vi "_Pull Controls Value to DPs(Refmgr).vi"(6 "sync DPs?(T)":bool=TRUE, 7 "VIRef(Caller VI)":refnum<k1>, 8 "error in (no error)":errorcluster, 9 "force update(F)":bool, 11 "SILAPI In":refnum<k1>) -> (0 "error out":errorcluster, 1 "Binded DPs":string[](array[string]), 3 "SILAPI Out":refnum<k1>)   [LabVIEW 2017, in "TagDB RefManager.lvlib"]
uses:
  TagDB RefManager.lvlib
  230c0da9-b6e4-44e0-8cb2-fe6bdec026ba.vi
  a90990ad-2366-4051-9646-140e847e3682.vi
  be640558-f0fc-44bb-96cd-108508b5fbdb.vi
  17cf8676-e257-4f33-957d-6af3ca117314.vi
  6c796322-1d76-4bdd-9aa2-7f47adde5471.vi
  024ec822-42c1-4cee-abf5-dbe2fbe4f70a.vi
  <userlib>/_NEVSTOP/TagDB/_Support/DataAccess/_NameCacher.vi
  <userlib>/_NEVSTOP/TagDB/_Support/Error/_[error50002]Invalid DataType.vi
  <userlib>/_NEVSTOP/TagDB/_Support/Error/_[error50000]Invalid DB REF.vi
  <userlib>/_NEVSTOP/TagDB/_Support/DataAccess/TagDB Ref to DVR.vi
  <userlib>/_NEVSTOP/TagDB/_Support/URL/TRIM-BOTH-SPACE.vi
  17cf8676-e257-4f33-957d-6af3ca117314.vi/1b47866c-8e2d-43a7-815f-8cf18635e5a1.vi
  6c796322-1d76-4bdd-9aa2-7f47adde5471.vi/1b47866c-8e2d-43a7-815f-8cf18635e5a1.vi
  <userlib>/_NEVSTOP/TagDB/_Support/DataAccess/data-Write.vi
  <userlib>/_NEVSTOP/TagDB/_Support/Change Detector/TagDB dbChanged.vi
  <userlib>/_NEVSTOP/TagDB/_Support/Error/_Clear Errors.vi
  17cf8676-e257-4f33-957d-6af3ca117314.vi/1b47866c-8e2d-43a7-815f-8cf18635e5a1.vi/29b2ea6d-6d7f-4e4a-ad31-a5cb760462c7.vi
  <userlib>/_NEVSTOP/TagDB/API/TagDB-Status.vi
  6c796322-1d76-4bdd-9aa2-7f47adde5471.vi/1b47866c-8e2d-43a7-815f-8cf18635e5a1.vi/29b2ea6d-6d7f-4e4a-ad31-a5cb760462c7.vi
  <userlib>/_NEVSTOP/TagDB/_Support/DataAccess/_datatypeChecker.vi
  <userlib>/_NEVSTOP/TagDB/_Support/Change Detector/TagDB ChangeFlag.vi
  <userlib>/_NEVSTOP/TagDB/_Support/Error/_Build Error Cluster.vi
  <vilib>/Utility/Data Type/Get Type Information.vi
  <userlib>/_NEVSTOP/TagDB/TagDB.lvlib
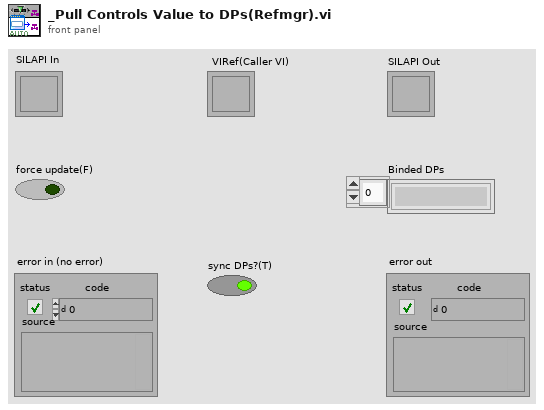
[diagram p1: front panel]
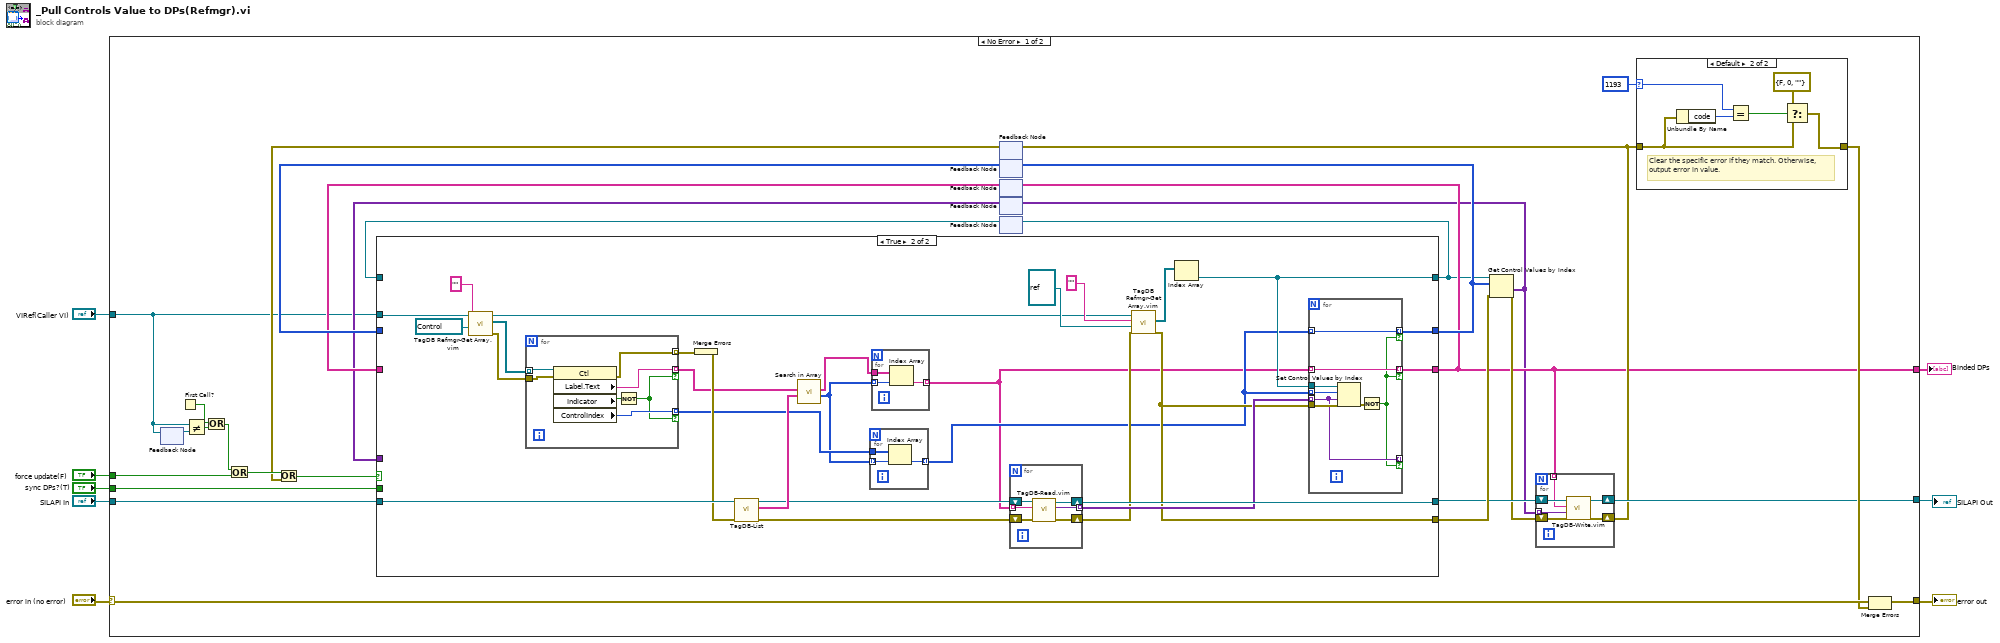
[diagram p0: block diagram]
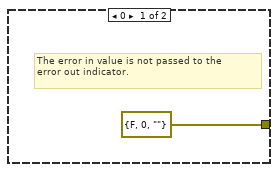
[diagram p2: hidden frame]
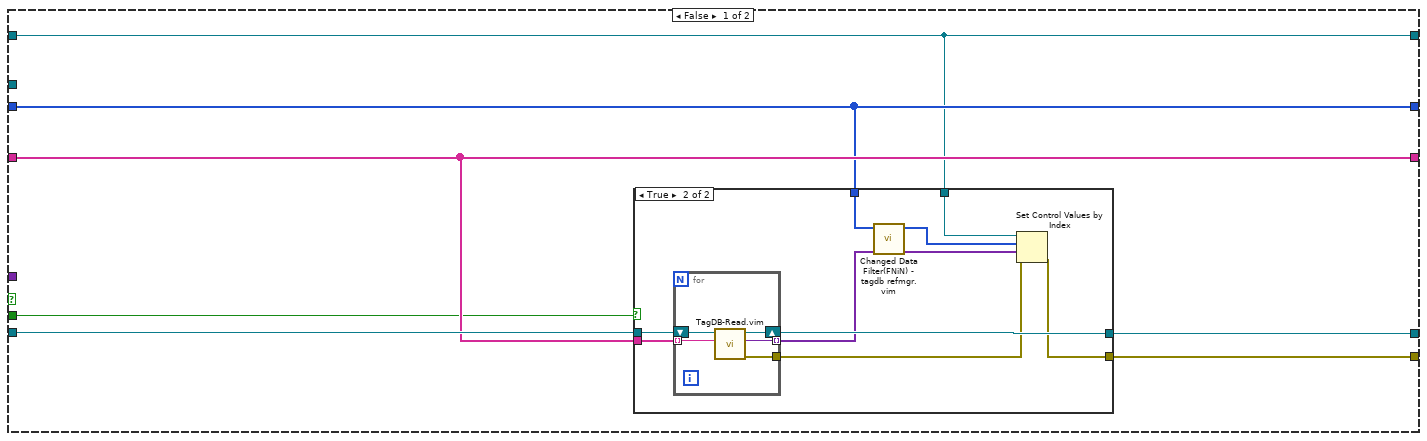
[diagram p3: hidden frame]
diagram:
  n1 = case shown="No Error" "error in (no error)" {
    selector: "error in (no error)" -> [w31 w129]
    tunnel: "force update(F)" -> [w36 _]
    tunnel: [w32 w129] -> w7
    tunnel: "SILAPI In" -> [w29 w128]
    tunnel: "VIRef(Caller VI)" -> [w9 _]
    tunnel: [w21 w128] -> w3
    tunnel: [w18 _] -> w2
    tunnel: "sync DPs?(T)" -> [w16 _]
    frame No Error {
      n2 = feedback #1() -> (w13:refnum<k1>)  [unwired: 1 in]
      n3 = feedback-in #1(w9) -> ()
      n4 = First Call?() -> (First Call?: T/F=w11:bool)
      n5 = Not Equal?(x=w9, y=w13) -> (x != y?=w12:bool)
      n6 = Or(x=w11, y=w12) -> (x .or. y?=w10:bool)
      n7 = Or(x=w10, y=w36) -> (x .or. y?=w33:bool)
      n8 = feedback #2() -> (w25:errorcluster)  [unwired: 1 in]
      n9 = Or(x=w33, y=w25) -> (x .or. y?=w26:bool)
      n10 = feedback #3() -> (w34:i32[])  [unwired: 1 in]
      n11 = feedback #4() -> (w30:string[])  [unwired: 1 in]
      n12 = feedback #5() -> (w28:variant[])  [unwired: 1 in]
      n13 = feedback #6() -> (w14:refnum<vi>)  [unwired: 1 in]
      n14 = case shown="True" w26 {
        tunnel: [w50 w80] -> w15
        tunnel: w9 -> [_ w88]
        tunnel: [w52 w95] -> w35
        tunnel: w34 -> [w52 _]
        tunnel: [w55 w96] -> w18
        tunnel: w30 -> [w55 _]
        tunnel: w29 -> [w56 w100]
        tunnel: [w53 w81] -> w23
        tunnel: w28 -> [_ _]
        tunnel: [w54 w98] -> w22
        tunnel: w16 -> [w51 _]
        tunnel: w14 -> [w50 _]
        frame False {
          n15 = case shown="True" w51 {
            tunnel: w56 -> [w57 w67]
            tunnel: w55 -> [_ w66]
            tunnel: [w57 w65] -> w54
            tunnel: w50 -> [_ w64]
            tunnel: [_ w62] -> w53
            tunnel: w52 -> [_ w59]
            frame False {
            }
            frame True {
              n16 = for {
                tunnel: w66 -> [w71] mode=indexing
                tunnel: [w69] -> w63
                tunnel: [w68] -> w61 mode=indexing
                shift-right: [w70] -> w65
                shift-left: w67 -> [w72]
                n17 = call "TagDB-Read.vim"("name"=w71, "TagDB"=w72) -> ("error out"=w69:errorcluster, "Value"=w68:variant, "TagDB(dup)"=w70:refnum<k1>)  [unwired: 4 in, 3 out]
              }
              n18 = call "Changed Data Filter(FNiN) - tagdb refmgr.vim"("checked data"=w61, "1"=w59) -> ("data"=w60:variant[], "1 out"=w58:i32[])  [unwired: 6 in, 2 out]
              n19 = Set Control Values by Index(0:w64, 1:w58, 2:w60, 3:w63) -> (11:w62:errorcluster)
            }
          }
        }
        frame True {
          n20 = call "TagDB Refmgr-Get Array.vim"("Type"=refnum<vi> refnum, "RegExp"="", "DB Ref"=w88) -> ("error out"=w87:errorcluster, "References"=w86:refnum<vi>[], "DB Ref(dup)"=w79:refnum<k1>)  [unwired: 5 in, 1 out]
          n21 = for {
            tunnel: w86 -> [w119] mode=indexing
            tunnel: [w118] -> w75 mode=indexing if=w113
            tunnel: [w117] -> w78 mode=indexing if=w113
            tunnel: [w115] -> w94 mode=indexing
            tunnel: w87 -> [w114]
            n22 = property class="Ctl"(reference=w119, error in=w114) -> (error out=w115:errorcluster, "Label.Text"=w118:string, "Indicator"=w116:bool, "ControlIndex"=w117:i32)  [unwired: 1 out]
            n23 = Not(x=w116) -> (.not. x?=w113:bool)
          }
          n24 = Merge Errors(w94) -> (w93:errorcluster)
          n25 = call <userlib>:"TagDB-List.vi"("error in (no error)"=w93, "TagDB"=w100) -> ("error out"=w99:errorcluster, "names"=w92:string[], "TagDB(dup)"=w91:refnum<k1>)  [unwired: 6 in, 1 out]
          n26 = call "Search in Array.vi"("items to filter"=w92, "array"=w75) -> ("item Indexs"=w76:i32[], "array(dup)"=w73:string[])  [unwired: 4 in]
          n27 = for {
            tunnel: w76 -> [w106] mode=indexing
            tunnel: w78 -> [w105]
            tunnel: [w104] -> w77 mode=indexing
            n28 = Index Array(array=w105, index=w106) -> (element=w104:i32)
          }
          n29 = for {
            tunnel: w76 -> [w103] mode=indexing
            tunnel: w73 -> [w102]
            tunnel: [w101] -> w74 mode=indexing
            n30 = Index Array(array=w102, index=w103) -> (element=w101:string)
          }
          n31 = for {
            tunnel: [w110] -> w97 mode=indexing
            tunnel: w74 -> [w108] mode=indexing
            shift-right: [w109] -> w82
            shift-left: w99 -> [w112]
            shift-right: [w111] -> w98
            shift-left: w91 -> [w107]
            n32 = call "TagDB-Read.vim"("error in (no error)"=w112, "name"=w108, "TagDB"=w107) -> ("error out"=w109:errorcluster, "Value"=w110:variant, "TagDB(dup)"=w111:refnum<k1>)  [unwired: 3 in, 3 out]
          }
          n33 = call "TagDB Refmgr-Get Array.vim"("error in (no error)"=w82, "Type"=refnum<vi> refnum ("Current VI Reference"), "RegExp"="", "DB Ref"=w79) -> ("error out"=w81:errorcluster, "References"=w83:refnum<vi>[])  [unwired: 4 in, 2 out]
          n34 = Index Array(array=w83) -> (element=w80:refnum<vi>)  [unwired: 1 in]
          n35 = for {
            tunnel: w80 -> [w127]
            tunnel: w77 -> [w126] mode=indexing
            tunnel: w97 -> [w122] mode=indexing
            tunnel: w81 -> [w125]
            tunnel: [w124] -> w96 mode=indexing if=w120
            tunnel: w74 -> [w124] mode=indexing
            tunnel: [w123] -> w95 mode=indexing if=w120
            tunnel: w77 -> [w123] mode=indexing
            tunnel: [w122] -> _ mode=indexing if=w120
            n36 = Set Control Values by Index(0:w127, 1:w126, 2:w122, 3:w125) -> (11:w121:errorcluster)
            n37 = Not(x=w121) -> (.not. x?=w120:bool)
          }
        }
      }
      n38 = feedback-in #3(w35) -> ()
      n39 = feedback-in #4(w18) -> ()
      n40 = feedback-in #6(w15) -> ()
      n41 = Get Control Values by Index(0:w15, 1:w35, 3:w23) -> (10:w17:variant[], 11:w20:errorcluster)
      n42 = feedback-in #5(w17) -> ()
      n43 = for {
        tunnel: w17 -> [w38] mode=indexing
        shift-right: [w41] -> w21
        shift-left: w22 -> [w42]
        shift-right: [w39] -> w19
        shift-left: w20 -> [w40]
        tunnel: w18 -> [w37] mode=indexing
        n44 = call "TagDB-Write.vim"("error in (no error)"=w40, "Value"=w38, "tag"=w37, "TagDB"=w42) -> ("error out"=w39:errorcluster, "TagDB(dup)"=w41:refnum<k1>)  [unwired: 5 in, 1 out]
      }
      n45 = feedback-in #2(w19) -> ()
      n46 = case shown="Default" 1193 ("specific error code to clear (0: all)") {
        selector: 1193 ("specific error code to clear (0: all)") -> [_ w48]
        tunnel: w19 -> [_ w47]
        tunnel: [errorcluster {"status"=FALSE, "code"=0, "source"=""} ("error constant") w44] -> w27
        frame 0 {
          # "The error in value is not passed to the\nerror out indicator."
        }
        frame Default {
          # "Clear the specific error if they match. Otherwise, output error in value."
          n47 = Unbundle By Name(w47) -> ("code"=w49:i32)
          n48 = Equal?(x=w48, y=w49) -> (x = y?=w45:bool)
          n49 = Select(t=errorcluster {"status"=FALSE, "code"=0, "source"=""} ("error constant"), s=w45, f=w47) -> (s? t:f=w44:errorcluster)
        }
      }
      n50 = Merge Errors(w31, w27) -> (w32:errorcluster)
    }
    frame Error {
    }
  }
  "error out" <- w7
  "SILAPI Out" <- w3
  "Binded DPs" <- w2
